vi "http.put_core.vi"(6 "specific headers in":cluster{"header":string, "value":string}[](array[cluster]), 8 "error in":errorcluster, 9 "Body":string, 10 "Path":string, 11 "REST Client":refnum<class "REST Client.lvclass">) -> (0 "error out":errorcluster, 2 "Response":string)   [LabVIEW 2020, in "Nominal Client.lvclass"]
uses:
  Nominal Client.lvclass
  <vilib>/addons/_JKI.lib/REST Client/classes/REST Client/REST Client.lvclass
  error.vi/859f8e04-e495-489b-b5b4-7ac163f56130.vi
  trace.calling_method.vi
  <vilib>/JDP Science/JDP Science Common Utilities/Trim Whitespace__JDP.vi
  <vilib>/AdvancedString/1D String Array to Delimited String.vi
  <vilib>/Utility/libraryn.llb/Get File Extension.vi
  log_file.write.vi
  <vilib>/JDP Science/JSONtext/Get all Object Items.vi
  <vilib>/Utility/error.llb/Error Cluster From Error Code.vi
  <vilib>/JDP Science/JSONtext/JSON text to Variant.vi
  <vilib>/JDP Science/JSONtext/LVClass Serializer/JSONtext LVClass Serializer.lvclass
  Nominal Client.lvclass/Nominal Client.ctl
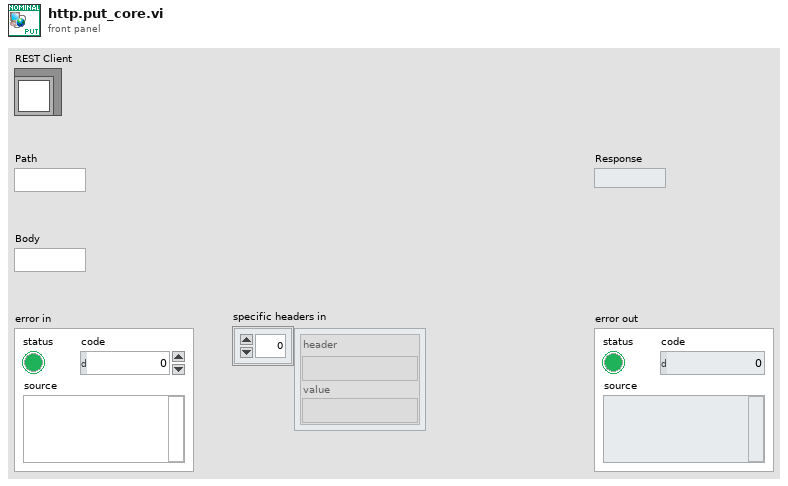
[diagram p1: front panel]
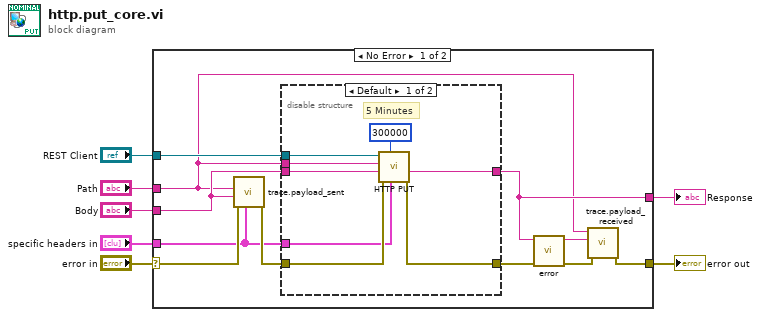
[diagram p0: block diagram]
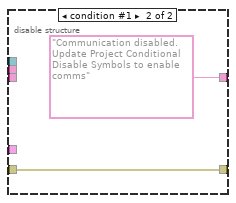
[diagram p2: hidden frame]
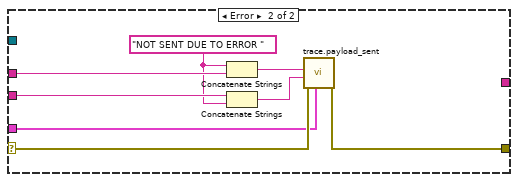
[diagram p3: hidden frame]
diagram:
  n1 = case shown="No Error" "error in" {
    selector: "error in" -> [w18 w31]
    tunnel: [w16 _] -> w7
    tunnel: "REST Client" -> [w14 _]
    tunnel: "Body" -> [w13 w34]
    tunnel: "specific headers in" -> [w12 w29]
    tunnel: [w8 w30] -> w2
    tunnel: "Path" -> [w10 w35]
    frame No Error {
      n2 = call "trace.payload_sent.vi"("Headers"=w12, "dataflow error in"=w18, "Request Body"=w13, "Path"=w10) -> ("dataflow error out"=w17:errorcluster)  [unwired: 7 in]
      n3 = disable-structure shown="Default" {
        disable-tunnel: [w26 "Communication disabled. Update Project Conditional Disable Symbols to enable comms" ("REST Response")] -> w16
        disable-tunnel: [w24 w28] -> w15
        disable-tunnel: w17 -> [w23 w28]
        disable-tunnel: w14 -> [w22 _]
        disable-tunnel: w13 -> [w21 _]
        disable-tunnel: w12 -> [w20 _]
        disable-tunnel: w10 -> [w19 _]
        frame condition #0 (active) {
          # "5 Minutes"
          n4 = call-dynamic "HTTP PUT.vi"("request specific headers"=w20, "timeout (0 = Use Default)"=300000, "error in (no error)"=w23, "Request body"=w21, "Path"=w19, "REST Client in"=w22) -> ("error out"=w24:errorcluster, "Response body"=w26:string)  [unwired: 4 out]
        }
        frame condition #1 {
        }
      }
      n5 = call "error.vi"("error in"=w15, "REST Response"=w16) -> ("error out"=w9:errorcluster, "Error Formatted Response"=w11:string)  [unwired: 8 in]
      n6 = call "trace.payload_received.vi"("dataflow error in"=w9, "Response"=w11, "Path"=w10) -> ("dataflow error out"=w8:errorcluster)  [unwired: 8 in]
    }
    frame Error {
      w33 = "NOT SENT DUE TO ERROR " ("string")
      n7 = Concatenate Strings(w33, w35) -> (w36:string)
      n8 = Concatenate Strings(w34, w33) -> (w32:string)
      n9 = call "trace.payload_sent.vi"("Headers"=w29, "dataflow error in"=w31, "Request Body"=w32, "Path"=w36) -> ("dataflow error out"=w30:errorcluster)  [unwired: 7 in]
    }
  }
  "error out" <- w2
  "Response" <- w7
